vi "Calc Row Stats.vi"(6 "Middle y":i32, 9 "Reciprocals":T2, 10 "Current Row":i32, 11 "Current Row":T1) -> (1 "Row width (pixels)":sgl, 3 "Next Row":T1, 5 "Start Col":i32, 7 "Number Of Cols This Row":i32)   [LabVIEW 2022 SP3, in "Raster.lvlib"]
uses:
  Raster.lvlib
  Reciprocals.ctl
  Current Row.ctl
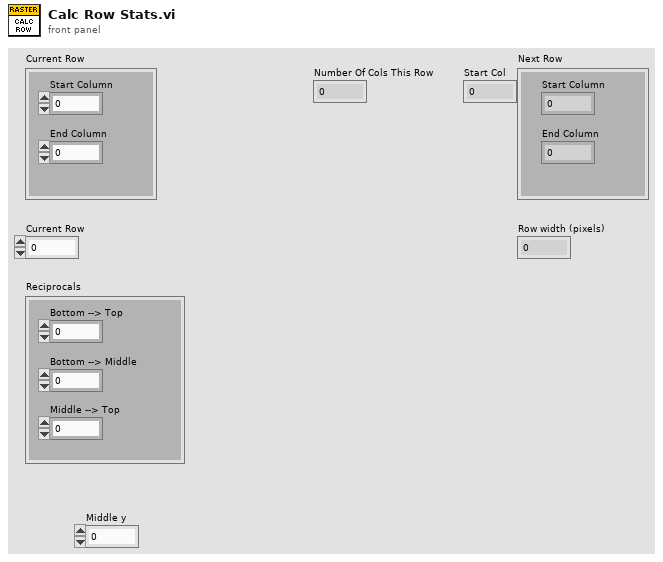
[diagram p1: front panel]
types:
  T1 = typedef "Raster.lvlib/Current Row.ctl" = cluster{"Start Column":sgl, "End Column":sgl}
  T2 = typedef "Raster.lvlib/Reciprocals.ctl" = cluster{"Bottom --> Top":sgl, "Bottom --> Middle":sgl, "Middle --> Top":sgl}
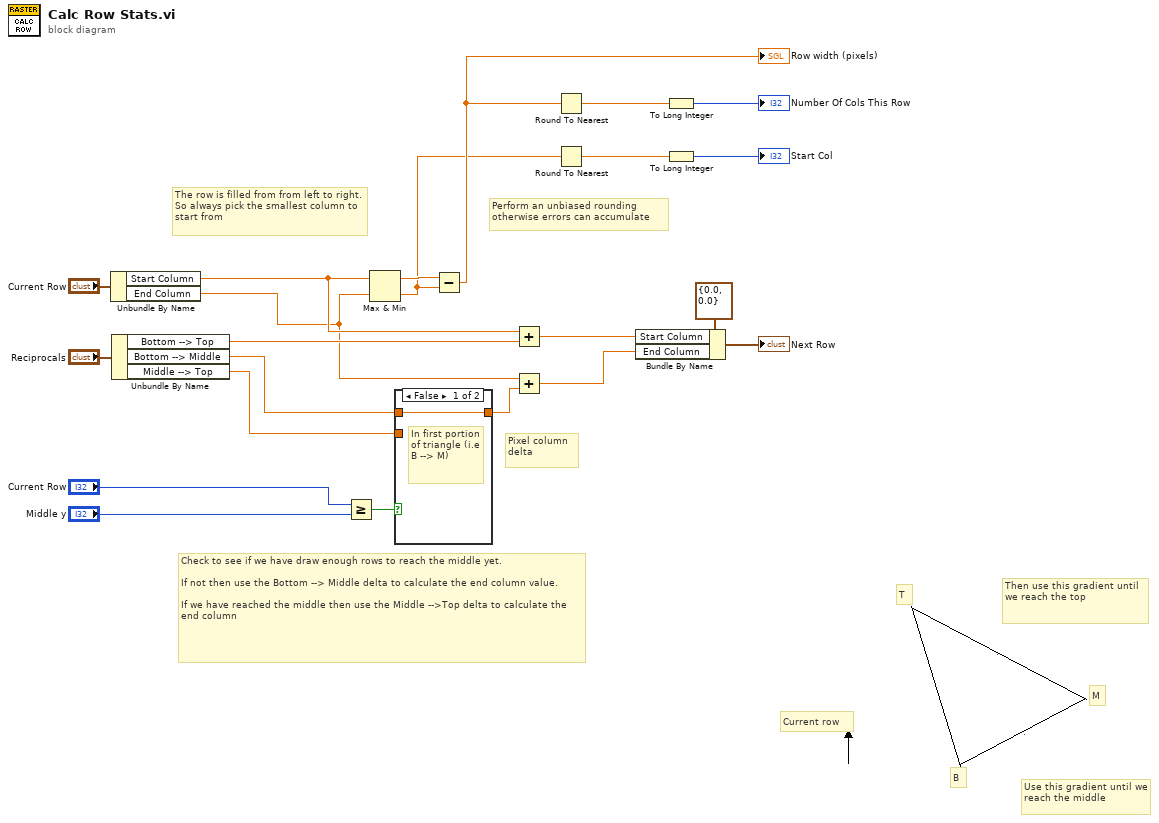
[diagram p0: block diagram]
diagram:
  # "."
  # "."
  # "Then use this gradient until we reach the top"
  # "Use this gradient until we reach the middle"
  # "Current row"
  # "M"
  # "T"
  # "B"
  # "Check to see if we have draw enough rows to reach the middle yet.\n\nIf not then use the Bottom --> Middle delta to calculate the end column value.\n\nIf we have reached the middle then use the Middle -->Top delta to calculate the end column"
  # "Perform an unbiased rounding otherwise errors can accumulate"
  # "The row is filled from from left to right. So always pick the smallest column to start from"
  # "Pixel column delta"
  n1 = Unbundle By Name("Current Row") -> ("Start Column"=w6:sgl, "End Column"=w5:sgl)
  n2 = Unbundle By Name("Reciprocals") -> ("Bottom --> Top"=w10:sgl, "Bottom --> Middle"=w9:sgl, "Middle --> Top"=w8:sgl)
  n3 = Greater Or Equal?(x="Current Row", y="Middle y") -> (x >= y?=w17:bool)
  n4 = Max & Min(x=w6, y=w5) -> (max(x,y)=w16:sgl, min(x,y)=w13:sgl)
  n5 = case shown="False" w17 {
    tunnel: w9 -> [w23 _]
    tunnel: [w23 w24] -> w15
    tunnel: w8 -> [_ w24]
    frame False {
      # "In first portion of triangle (i.e B --> M)"
    }
    frame True {
      # "In second portion of triangle (i.e M --> T)"
    }
  }
  n6 = Subtract(x=w16, y=w13) -> (x-y=w22:sgl)
  "Row width (pixels)" <- w22
  n7 = Add(x=w6, y=w10) -> (x+y=w2:sgl)
  n8 = Add(x=w5, y=w15) -> (x+y=w1:sgl)
  n9 = Round To Nearest(number=w22) -> (nearest integer value=w21:sgl)
  n10 = Round To Nearest(number=w13) -> (nearest integer value=w12:sgl)
  n11 = Bundle By Name(cluster=T1 {"Start Column"=0.0, "End Column"=0.0} ("Current Row"), "Start Column"=w2, "End Column"=w1) -> (→"Next Row":T1)
  n12 = To Long Integer(number=w21) -> (32bit integer=→"Number Of Cols This Row":i32)
  n13 = To Long Integer(number=w12) -> (32bit integer=→"Start Col":i32)
